vi "Build Array.vi"() -> ()   [LabVIEW 2023]
doc: "This example shows how the Build Array function operates in two different modes: concatenate and append. This example only shows numeric arrays, but the same functionality exists for any array type."
panel:
  out "Appended Array":i32[][](array[numeric])
  out "Concatenated Array":i32[](array[numeric])
  in  "Array of Numeric Data 3":i32[](array[numeric])=[5, 6, 7]
  in  "Array of Numeric Data 2":i32[](array[numeric])=[2, 3, 4]
  in  "Array of Numeric Data 1":i32[](array[numeric])=[1]
  # "Overview: Demonstrates how the Build Array function operates in two modes: concatenate and append.\nInstructions:\n1. Run the VI.\n2. Examine the different cases."
  # "In Concatenate Inputs Mode, the Build Array function appends all inputs in order, forming an output array of the same dimensionality as the array input wired."
  # "If the Build Array function is not in Concatenate Mode, it is in Append Mode.  In Append Mode, the Build Array function creates an array of one dimension higher than the dimension of the inputs. All the inputs must be the same dimensionality.  The array will be padded with default values when the inputs differ in size."
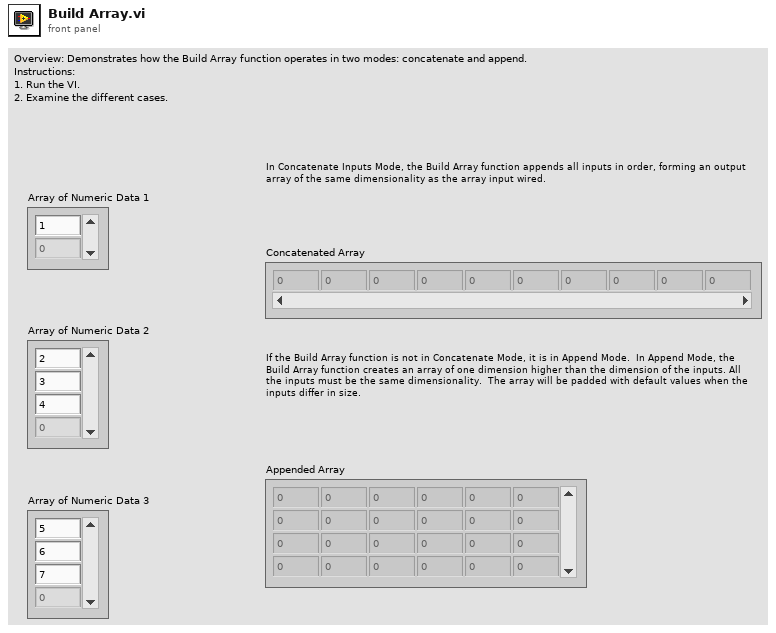
[diagram p1: front panel]
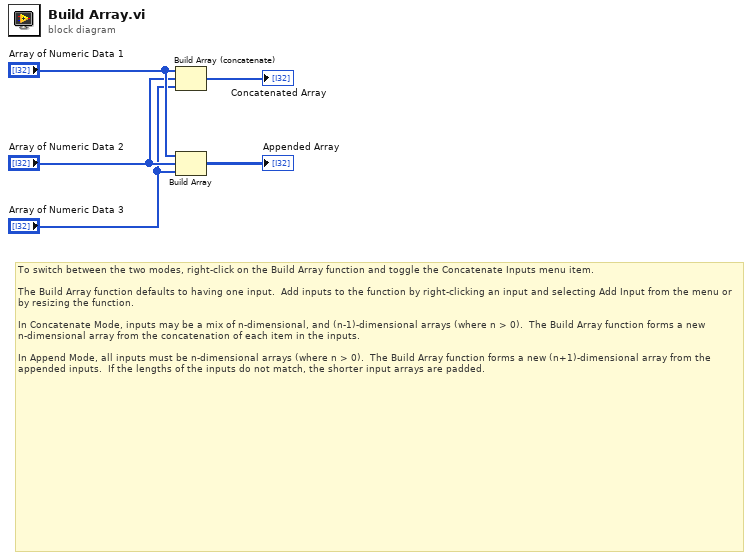
[diagram p0: block diagram]
diagram:
  # "To switch between the two modes, right-click on the Build Array function and toggle the Concatenate Inputs menu item.\n\nThe Build Array function defaults to having one input.  Add inputs to the function by right-clicking an input and selecting Add Input from the menu or by resizing the function.\n\nIn Concatenate Mode, inputs may be a mix of n-dimensional, and (n-1)-dimensional arrays (where n > 0).  The Build Array function forms a new n-dimensional array from the concatenation of each item in the inputs.\n\nIn Append Mode, all inputs must be n-dimensional arrays (where n > 0).  The Build Array function forms a new (n+1)-dimensional array from the appended inputs.  If the lengths of the inputs do not match, the shorter input arrays are padded."
  n1 = Build Array (concatenate)("Array of Numeric Data 1", "Array of Numeric Data 2", "Array of Numeric Data 3") -> (→"Concatenated Array":i32[])
  n2 = Build Array("Array of Numeric Data 1", "Array of Numeric Data 2", "Array of Numeric Data 3") -> (→"Appended Array":i32[][])
